vi "Post - SGL Array.vi"(6 "timestamp":timestamp, 7 "PV name":string, 8 "error in (no error)":errorcluster, 10 "value":sgl[](array[numeric]), 11 "Server in":refnum<class "Server.lvclass">) -> (0 "error out":errorcluster, 3 "Server out":refnum<class "Server.lvclass">)   [LabVIEW 2020, in "PV Access.lvlib" / "PVA Server.lvlib" / "Server.lvclass"]
uses:
  Server.lvclass
  Server.lvclass/Server.ctl
  25a0afa2-78cc-4e41-9cb9-729b0faefda4.vi
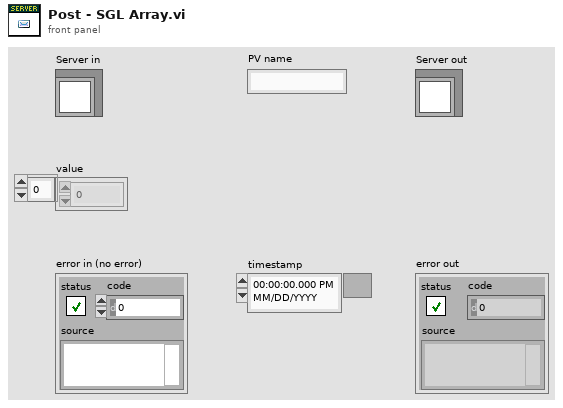
[diagram p1: front panel]
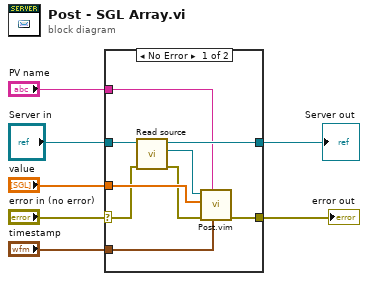
[diagram p0: block diagram]
diagram:
  n1 = case shown="No Error" "error in (no error)" {
    selector: "error in (no error)" -> [w10 w18]
    tunnel: [w11 w18] -> w2
    tunnel: [w15 w17] -> w1
    tunnel: "Server in" -> [w16 w17]
    tunnel: "PV name" -> [w12 _]
    tunnel: "value" -> [w14 _]
    tunnel: "timestamp" -> [w8 _]
    frame No Error {
      n2 = call "Read source.vi"("error in (no error)"=w10, "Server in"=w16) -> ("error out"=w9:errorcluster, "Source"=w13:refnum<class "Source.lvclass">, "Server out"=w15:refnum<class "Server.lvclass">)  [unwired: 7 in]
      n3 = call "Post.vim"("timestamp"=w8, "PV name"=w12, "error in"=w9, "value"=w14, "Source in"=w13) -> ("error out"=w11:errorcluster)  [unwired: 5 in, 1 out]
    }
    frame Error {
    }
  }
  "error out" <- w2
  "Server out" <- w1
